vi "Cache_Members Load.vi"(8 "error in (no error)":errorcluster, 10 "Class Name":string, 11 "Refnum in":T1) -> (0 "error out":errorcluster, 1 "Success?":bool, 2 "Member Map":T2, 3 "Refnum out":T1)   [LabVIEW 2019, in "ClassLoader.lvlib"]
uses:
  ClassLoader.lvlib
  <vilib>/Utility/config.llb/NI_LVConfig.lvlib
  <vilib>/Utility/Data Type/Member VI Info.ctl
  Ctl/Ctl_Member Map.ctl
  <vilib>/Utility/config.llb/Config Data RefNum.ctl
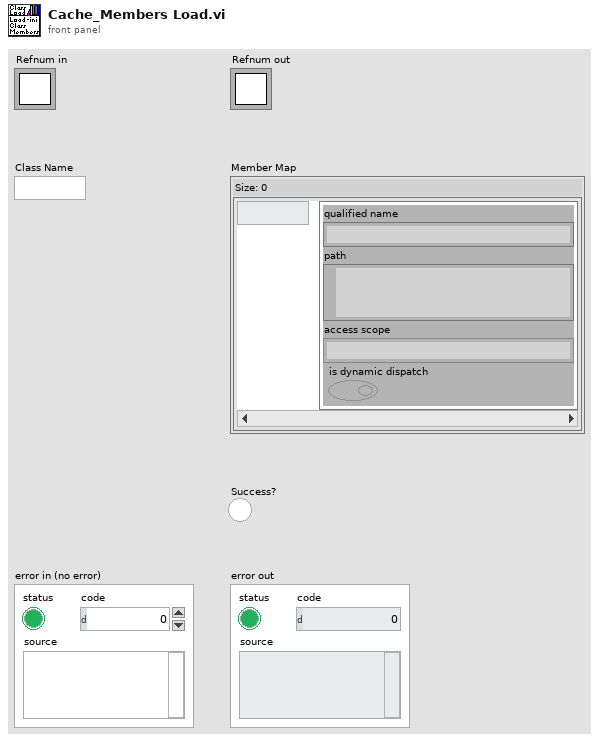
[diagram p1: front panel]
types:
  T1 = typedef "NI_LVConfig.lvlib/Config Data RefNum.ctl" = refnum<k1>
  T2 = typedef "ClassLoader.lvlib/Ctl_Member Map.ctl" = map{string, T3}
  T3 = typedef "Member VI Info.ctl" = cluster{"qualified name":string, "path":path, "access scope":enum32{"invalid scope", "public", "private", "protected", "community"}, "is dynamic dispatch":bool}
  T4 = enum32{"invalid scope", "public", "private", "protected", "community"}
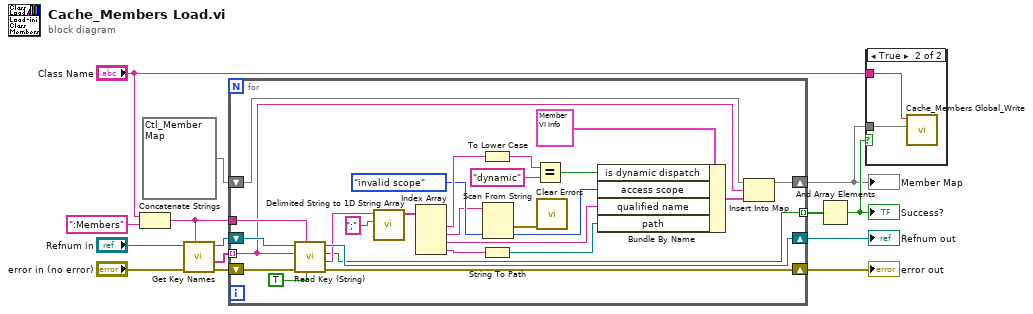
[diagram p0: block diagram]
diagram:
  n1 = Concatenate Strings("Class Name", ":Members" ("string")) -> (w7:string)
  n2 = call <vilib>:"Get Key Names.vi"("section"=w7, "error in (no error)"="error in (no error)", "refnum"="Refnum in") -> ("error out"=w5:errorcluster, "key names"=w6:string[], "refnum out"=w4:T1)  [unwired: 5 in, 1 out]
  n3 = for {
    shift-right: [w37] -> w8
    shift-left: w4 -> [w40]
    shift-right: [w36] -> w9
    shift-left: w5 -> [w39]
    tunnel: w6 -> [w18] mode=indexing
    tunnel: w7 -> [w38]
    shift-right: [w19] -> w13
    shift-left: T2 {} ("Member Map") -> [w20]
    tunnel: [w16] -> w10 mode=indexing
    n4 = call <vilib>:"Read Key (String).vi"("read raw string? (F)"=TRUE, "section"=w38, "error in (no error)"=w39, "key"=w18, "refnum"=w40) -> ("error out"=w36:errorcluster, "value"=w34:string, "found?"=w16:bool, "refnum out"=w37:T1)  [unwired: 3 in]
    n5 = call <vilib>:"Delimited String to 1D String Array.vi"("delimiter"=";", "delimited string"=w34) -> ("string array"=w32:string[])  [unwired: 9 in]
    n6 = Index Array(array=w32) -> (element #1=w31:string, element #2=w26:string, element #3=w23:string, element #4=w22:string)  [unwired: 4 in]
    n7 = To Lower Case(string=w31) -> (all lower case string=w30:string)
    n8 = String To Path(string=w22) -> (path=w21:path)
    n9 = Scan From String(input string=w26, default 1=T4."invalid scope" ("access scope")) -> (error out=w24:errorcluster, output 1=w25:T4)  [unwired: 3 in, 2 out]
    n10 = Equal?(x=w30, y="dynamic") -> (x = y?=w28:bool)
    n11 = call <vilib>:"Clear Errors.vi"("error in (no error)"=w24) -> ()  [unwired: 5 in, 2 out]
    n12 = Bundle By Name(cluster=T3 {"qualified name"="", "path"=path "", "access scope"=enum."invalid scope", "is dynamic dispatch"=FALSE} ("VI info"), "is dynamic dispatch"=w28, "access scope"=w25, "qualified name"=w23, "path"=w21) -> (w17:T3)
    n13 = Insert Into Map(map in=w20, key=w18, value=w17) -> (map out=w19:T2)  [unwired: 2 out]
  }
  "Member Map" <- w13
  "error out" <- w9
  "Refnum out" <- w8
  n14 = And Array Elements(Boolean array=w10) -> (logical AND=w14:bool)
  "Success?" <- w14
  n15 = case shown="True" w14 {
    tunnel: "Class Name" -> [_ w42]
    tunnel: w13 -> [_ w41]
    frame False {
    }
    frame True {
      n16 = call "Cache_Members Global_Write.vi"("Member Map"=w41, "Class Name"=w42) -> ()  [unwired: 10 in]
    }
  }
